vi "EI (A).vi"(0 "Sampler":refnum<k24>, 1 "Ei":refnum<k24>, 2 "CellOnOff":i32(ring) items=["Off", "On"], 3 "Setpoint":dbl, 4 "Bandwidth":i32(ring)=2 items=["UltraHigh_Speed", "High_Speed", "High_Stability"], 5 "CurrentRange":i32(ring)=-3 items=["CR07_1A"=0, "CR06_10A"=1, "CR01_100A"=2, "CR00_1000A"=3, "CR05_20A"=20, "CR04_40A"=40, "CR03_50A"=60, "CR02_80A"=80, "CR19_1pA"=-12, "CR18_10pA"=-11, "CR17_100pA"=-10, "CR16_1nA"=-9, "CR15_10nA"=-8, "CR14_100nA"=-7, "CR13_1uA"=-6, "CR12_10uA"=-5, "CR11_100uA"=-4, "CR10_1mA"=-3, "CR09_10mA"=-2, "CR08_100mA"=-1], 6 "Mode":i32(ring) items=["Potentiostatic", "Galvanostatic"], 7 "error in (no error)":errorcluster, 8 "Disable Sampler":bool) -> (14 "Cell":bool, 15 "PotentialOverload":bool, 16 "ManualCellSwitch":bool, 17 "TemperatureOverload":bool, 18 "CurrentOverload":bool, 19 "Oscillation":bool, 20 "Setpoint":dbl, 21 "Bandwidth":i32(ring) items=["UltraHigh_Speed", "High_Speed", "High_Stability"], 22 "CurrentRange":i32(ring) items=["CR07_1A"=0, "CR06_10A"=1, "CR01_100A"=2, "CR00_1000A"=3, "CR05_20A"=20, "CR04_40A"=40, "CR03_50A"=60, "CR02_80A"=80, "CR19_1pA"=-12, "CR18_10pA"=-11, "CR17_100pA"=-10, "CR16_1nA"=-9, "CR15_10nA"=-8, "CR14_100nA"=-7, "CR13_1uA"=-6, "CR12_10uA"=-5, "CR11_100uA"=-4, "CR10_1mA"=-3, "CR09_10mA"=-2, "CR08_100mA"=-1], 23 "Mode":i32(ring) items=["Potentiostatic", "Galvanostatic"], 24 "EI status supported for":string[](array[string]), 25 "Potential":dbl, 26 "Current":dbl, 27 "error out":errorcluster)   [LabVIEW 2020]
doc: "Electrochemical Interface control panel (advanced version). For some autolabs not all properties are available, check the \"EI status supported for\" which properties are available for the connected instrument."
uses:
  C:/Users/Benj/Desktop/SEC Software V4.9/EcoChemie.Autolab.Sdk.dll
  SEC Software V4.9/EcoChemie.Autolab.Sdk.dll
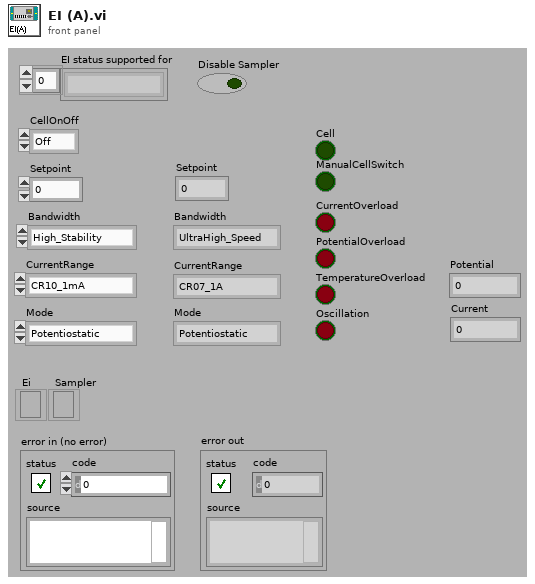
[diagram p1: front panel]
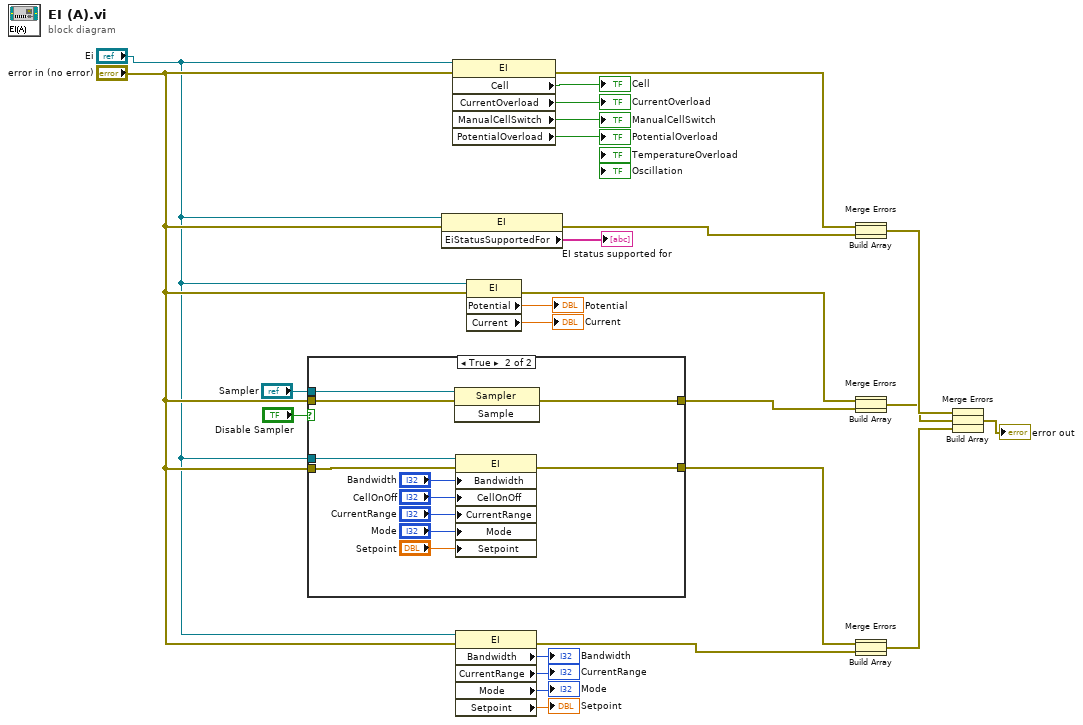
[diagram p0: block diagram]
diagram:
  n1 = case shown="True" "Disable Sampler" {
    tunnel: [w31 w42] -> w22
    tunnel: "error in (no error)" -> [w31 w41]
    tunnel: "Ei" -> [_ w36]
    tunnel: "error in (no error)" -> [w30 w35]
    tunnel: "Sampler" -> [_ w33]
    tunnel: [w30 w32] -> w13
    frame False {
    }
    frame True {
      n2 = invoke class="Sampler" method="Sample"(reference=w33, error in=w41) -> (error out=w42:errorcluster)  [unwired: 1 in, 2 out]
      n3 = property class="EI"(reference=w36, error in=w35, "Bandwidth"="Bandwidth", "CellOnOff"="CellOnOff", "CurrentRange"="CurrentRange", "Mode"="Mode", "Setpoint"="Setpoint") -> (error out=w32:errorcluster)  [unwired: 1 out]
    }
  }
  n4 = property class="EI"(reference="Ei", error in="error in (no error)") -> (error out=w16:errorcluster, "EiStatusSupportedFor"=→"EI status supported for":string[])  [unwired: 1 out]
  n5 = property class="EI"(reference="Ei", error in="error in (no error)") -> (error out=w15:errorcluster, "Cell"=→"Cell":bool, "CurrentOverload"=→"CurrentOverload":bool, "ManualCellSwitch"=→"ManualCellSwitch":bool, "PotentialOverload"=→"PotentialOverload":bool)  [unwired: 1 out]
  n6 = property class="EI"(reference="Ei", error in="error in (no error)") -> (error out=w14:errorcluster, "Bandwidth"=→"Bandwidth":i32, "CurrentRange"=→"CurrentRange":i32, "Mode"=→"Mode":i32, "Setpoint"=→"Setpoint":dbl)  [unwired: 1 out]
  n7 = property class="EI"(reference="Ei", error in="error in (no error)") -> (error out=w23:errorcluster, "Potential"=→"Potential":dbl, "Current"=→"Current":dbl)  [unwired: 1 out]
  n8 = Build Array(w15, w16) -> (w1:errorcluster[])
  n9 = Merge Errors(w1) -> (w12:errorcluster)
  n10 = Build Array(w23, w22) -> (w4:errorcluster[])
  n11 = Merge Errors(w4) -> (w11:errorcluster)
  n12 = Build Array(w13, w14) -> (w2:errorcluster[])
  n13 = Merge Errors(w2) -> (w10:errorcluster)
  n14 = Build Array(w12, w11, w10) -> (w3:errorcluster[])
  n15 = Merge Errors(w3) -> (→"error out":errorcluster)
